vi "MaxiGauge_Error.vi"() -> ()   [LabVIEW 2019]
panel:
  in  "stop":bool
  out "Sensor":string
  out "Output 2":string
  in  "Delay":u32=500
  in  "VISA resource name":refnum<visa-resource-name>
  out "Output 1":string
  out "System":string
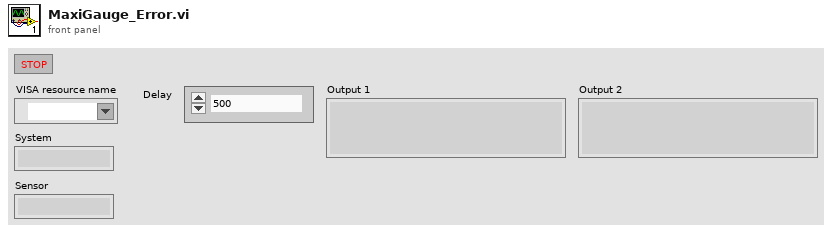
[diagram p1: front panel]
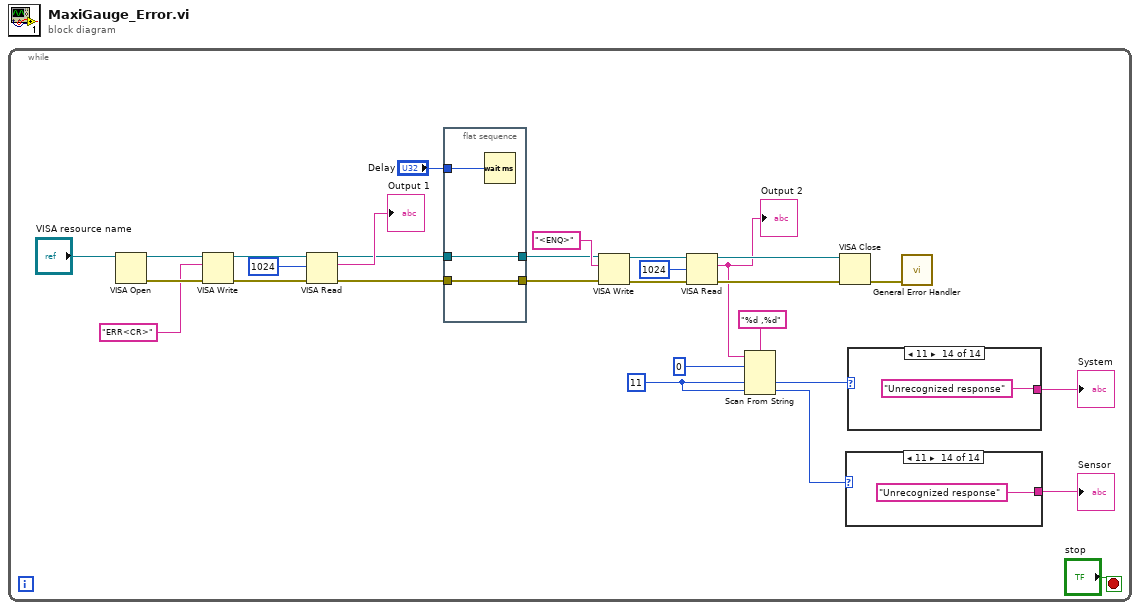
[diagram p0: block diagram]
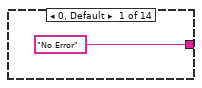
[diagram p2: hidden frame]
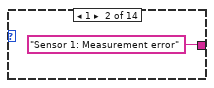
[diagram p3: hidden frame]
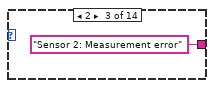
[diagram p4: hidden frame]
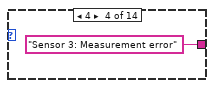
[diagram p5: hidden frame]
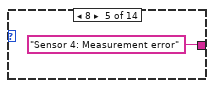
[diagram p6: hidden frame]
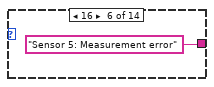
[diagram p7: hidden frame]
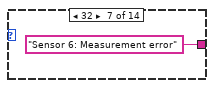
[diagram p8: hidden frame]
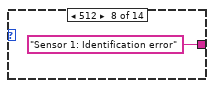
[diagram p9: hidden frame]
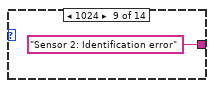
[diagram p10: hidden frame]
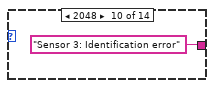
[diagram p11: hidden frame]
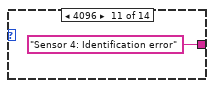
[diagram p12: hidden frame]
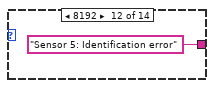
[diagram p13: hidden frame]
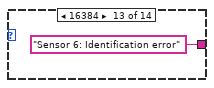
[diagram p14: hidden frame]
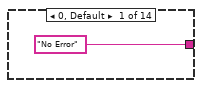
[diagram p15: hidden frame]
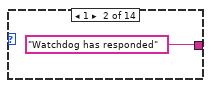
[diagram p16: hidden frame]
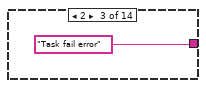
[diagram p17: hidden frame]
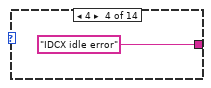
[diagram p18: hidden frame]
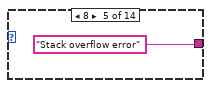
[diagram p19: hidden frame]
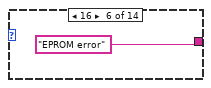
[diagram p20: hidden frame]
diagram:
  n1 = while {
    stop <- "stop" stop-if-true
    w2 = u32 11 ("unsigned 32bit integer")
    n2 = VISA Open(VISA resource name="VISA resource name") -> (VISA resource name=w28:refnum<visa-resource-name>, error out=w26:errorcluster)  [unwired: 4 in]
    n3 = VISA Write(VISA resource name=w28, write buffer="ERR<CR>" ("String"), error in (no error)=w26) -> (VISA resource name out=w27:refnum<visa-resource-name>, error out=w25:errorcluster)  [unwired: 1 out]
    n4 = VISA Read(VISA resource name=w27, byte count=u32 1024 ("unsigned 32bit integer"), error in (no error)=w25) -> (VISA resource name out=w14:refnum<visa-resource-name>, read buffer=→"Output 1":string, error out=w12:errorcluster)  [unwired: 1 out]
    n5 = flat-sequence {
      tunnel: "Delay" -> [w60]
      tunnel: [w59] -> w13
      tunnel: w14 -> [w59]
      tunnel: [w58] -> w11
      tunnel: w12 -> [w58]
      frame #0 {
        n6 = Wait (ms)(milliseconds to wait=w60) -> ()  [unwired: 1 out]
      }
    }
    n7 = VISA Write(VISA resource name=w13, write buffer="<ENQ>" ("String"), error in (no error)=w11) -> (VISA resource name out=w23:refnum<visa-resource-name>, error out=w21:errorcluster)  [unwired: 1 out]
    n8 = VISA Read(VISA resource name=w23, byte count=u32 1024 ("unsigned 32bit integer"), error in (no error)=w21) -> (VISA resource name out=w17:refnum<visa-resource-name>, read buffer=w8:string, error out=w19:errorcluster)  [unwired: 1 out]
    "Output 2" <- w8
    n9 = Scan From String(format string="%d ,%d", input string=w8, initial scan location=u32 0 ("unsigned 32bit integer"), default 1=w2, default 2=w2) -> (output 1=w6:u32, output 2=w4:u32)  [unwired: 1 in, 3 out]
    n10 = VISA Close(VISA resource name=w17, error in (no error)=w19) -> (error out=w16:errorcluster)
    n11 = case shown="11" w4 {
      tunnel: ["No Error" ("String") "Sensor 1: Measurement error" ("String") "Sensor 2: Measurement error" ("String") "Sensor 3: Measurement error" ("String") "Sensor 4: Measurement error" ("String") "Sensor 5: Measurement error" ("String") "Sensor 6: Measurement error" ("String") "Sensor 1: Identification error" ("String") "Sensor 2: Identification error" ("String") "Sensor 3: Identification error" ("String") "Sensor 4: Identification error" ("String") "Sensor 5: Identification error" ("String") "Sensor 6: Identification error" ("String") "Unrecognized response" ("String")] -> w3
      frame 0, Default {
      }
      frame 1 {
      }
      frame 2 {
      }
      frame 4 {
      }
      frame 8 {
      }
      frame 16 {
      }
      frame 32 {
      }
      frame 512 {
      }
      frame 1024 {
      }
      frame 2048 {
      }
      frame 4096 {
      }
      frame 8192 {
      }
      frame 16384 {
      }
      frame 11 {
      }
    }
    "Sensor" <- w3
    n12 = case shown="11" w6 {
      tunnel: ["No Error" ("String") "Watchdog has responded" ("String") "Task fail error" ("String") "IDCX idle error" ("String") "Stack overflow error" ("String") "EPROM error" ("String") "RAM error" ("String") "EEPROM error" ("String") "Key error" ("String") "Syntax error" ("String") "Inadmissible parameter" ("String") "No hardware" ("String") "Fatal error" ("String") "Unrecognized response" ("String")] -> w5
      frame 0, Default {
      }
      frame 1 {
      }
      frame 2 {
      }
      frame 4 {
      }
      frame 8 {
      }
      frame 16 {
      }
      frame 32 {
      }
      frame 64 {
      }
      frame 128 {
      }
      frame 4096 {
      }
      frame 8192 {
      }
      frame 16384 {
      }
      frame 32768 {
      }
      frame 11 {
      }
    }
    "System" <- w5
    n13 = call <vilib>:"General Error Handler.vi"("error in (no error)"=w16) -> ()  [unwired: 10 in, 5 out]
  }
